vi "PH_Strings.Seconds out of Clockstring.vi"(1 "Clock String":string) -> (0 "Time [s]":dbl)   [LabVIEW 2014, in "PH_Common.lvlib"]
doc: "This VI calculates seconds out of a clockstring of the form HH:MM:ss, MM:ss or s."
uses:
  PH_Common.lvlib
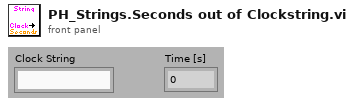
[diagram p1: front panel]
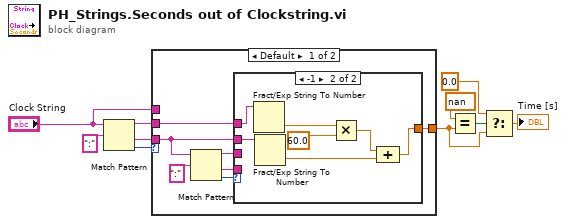
[diagram p0: block diagram]
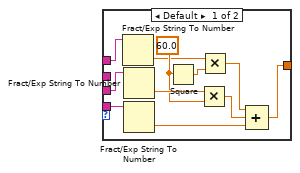
[diagram p2: hidden frame]
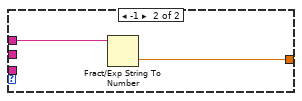
[diagram p3: hidden frame]
diagram:
  n1 = Match Pattern(string="Clock String", regular expression=":") -> (before substring=w9:string, after substring=w10:string, offset past match=w2:i32)  [unwired: 1 in, 1 out]
  n2 = case shown="Default" w2 {
    tunnel: "Clock String" -> [_ w37]
    tunnel: [w16 w36] -> w8
    tunnel: w9 -> [w17 _]
    tunnel: w10 -> [w15 _]
    frame Default {
      n3 = Match Pattern(string=w15, regular expression=":") -> (before substring=w12:string, after substring=w11:string, offset past match=w13:i32)  [unwired: 1 in, 1 out]
      n4 = case shown="-1" w13 {
        tunnel: w17 -> [w28 w35]
        tunnel: [w18 w32] -> w16
        tunnel: w15 -> [_ w29]
        tunnel: w12 -> [w23 _]
        tunnel: w11 -> [w22 _]
        frame Default {
          w26 = 60.0 ("y")
          n5 = Fract/Exp String To Number(string=w28) -> (number=w25:dbl)  [unwired: 3 in, 1 out]
          n6 = Fract/Exp String To Number(string=w23) -> (number=w27:dbl)  [unwired: 3 in, 1 out]
          n7 = Fract/Exp String To Number(string=w22) -> (number=w19:dbl)  [unwired: 3 in, 1 out]
          n8 = Square(x=w26) -> (x^2=w24:dbl)
          n9 = Multiply(x=w27, y=w26) -> (x*y=w20:dbl)
          n10 = Multiply(x=w25, y=w24) -> (x*y=w21:dbl)
          n11 = Compound Arithmetic op=ADD(w21, w20, w19) -> (w18:dbl)
        }
        frame -1 {
          n12 = Fract/Exp String To Number(string=w35) -> (number=w34:dbl)  [unwired: 3 in, 1 out]
          n13 = Fract/Exp String To Number(string=w29) -> (number=w30:dbl)  [unwired: 3 in, 1 out]
          n14 = Multiply(x=w34, y=60.0) -> (x*y=w33:dbl)
          n15 = Compound Arithmetic op=ADD(w33, w30) -> (w32:dbl)
        }
      }
    }
    frame -1 {
      n16 = Fract/Exp String To Number(string=w37) -> (number=w36:dbl)  [unwired: 3 in, 1 out]
    }
  }
  n17 = Equal?(x=nan ("y"), y=w8) -> (x = y?=w4:bool)
  n18 = Select(t=0.0, s=w4, f=w8) -> (s? t:f=→"Time [s]":dbl)
